vi "StartPlayRslt.vi"(8 "error in (no error)":errorcluster, 11 "CameraTestingENI":refnum<class "CameraTestingENI.lvclass">) -> (0 "error out":errorcluster, 3 "CameraTestingENI":refnum<class "CameraTestingENI.lvclass">)   [LabVIEW 2020, in "CameraTestingProxy.lvlib" / "CameraTestingENI.lvclass"]
uses:
  CameraTestingENI.lvclass
  CameraTestingENI.lvclass/CameraTestingENI.ctl
  e741e379-9b6b-4226-98e1-91cb9680b391.vi
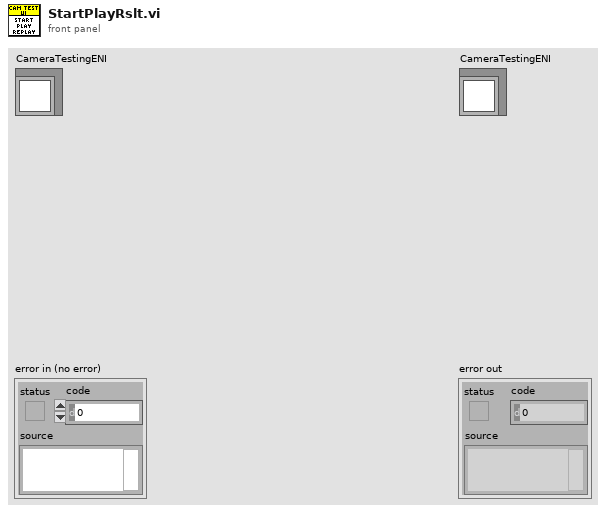
[diagram p1: front panel]
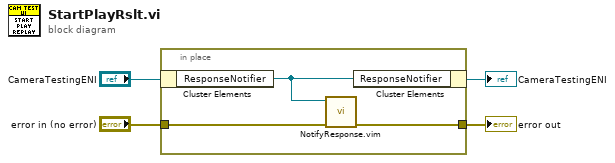
[diagram p0: block diagram]
diagram:
  n1 = in-place {
    in-place-border: "error in (no error)" -> [w7]
    in-place-border: [w5] -> w1
    n2 = in-place-cluster #1("CameraTestingENI") -> ("ResponseNotifier"=w6:refnum<notifier>)
    n3 = call "NotifyResponse.vim"("error in (no error)"=w7, "ResponseNotifier"=w6) -> ("error out"=w5:errorcluster)  [unwired: 9 in]
    n4 = in-place-cluster #1("ResponseNotifier"=w6) -> (→"CameraTestingENI":refnum<class "CameraTestingENI.lvclass">)
  }
  "error out" <- w1
